vi "Reorder View to Direction.vi"(10 "View in":i32[](array[numeric]), 11 "Primary Direction":T1) -> (2 "View out":i32[](array[numeric]), 3 "Direction List":T1[](array[typedef]))   [LabVIEW 2017, in "AntFarm_MB.lvclass"]
uses:
  AntFarm_MB.lvclass
  Type Defs/Direction Enum.ctl
  Type Defs/SB Type Defs.lvlib
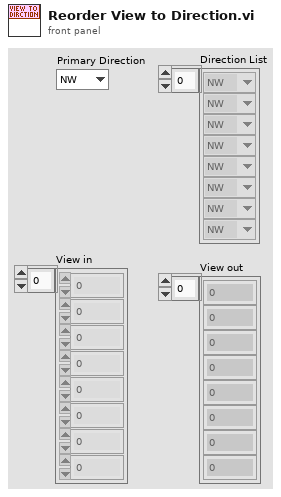
[diagram p1: front panel]
types:
  T1 = typedef "SB Type Defs.lvlib/Direction Enum.ctl" = enum16{"NW", "N", "NE", "E", "SE", "S", "SW", "W"}
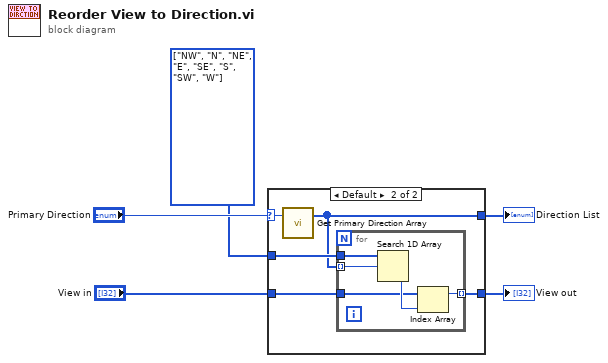
[diagram p0: block diagram]
diagram:
  w1 = T1[] [enum."NW", enum."N", enum."NE", enum."E", enum."SE", enum."S", enum."SW", enum."W"] items=["NW", "N", "NE", "E", "SE", "S", "SW", "W"]
  n1 = case shown="Default" "Primary Direction" {
    selector: "Primary Direction" -> [_ w12]
    tunnel: w1 -> [w7 w11]
    tunnel: [w7 w9] -> w3
    tunnel: "View in" -> [w6 w10]
    tunnel: [w6 w8] -> w5
    frame "NW" {
    }
    frame Default {
      n2 = call "Get Primary Direction Array.vi"("Primary Direction"=w12) -> ("Direction Array"=w9:T1[])  [unwired: 2 in]
      n3 = for {
        tunnel: w11 -> [w17]
        tunnel: w9 -> [w16] mode=indexing
        tunnel: w10 -> [w14]
        tunnel: [w13] -> w8 mode=indexing
        n4 = Search 1D Array(1D array=w17, element=w16) -> (index of element=w15:i32)  [unwired: 1 in]
        n5 = Index Array(array=w14, index=w15) -> (element=w13:i32)
      }
    }
  }
  "View out" <- w5
  "Direction List" <- w3
